vi "Test_Move_Relative.vi"() -> ()   [LabVIEW 2019]
panel:
  in  "Speed input":i16
  in  "Acceleration input":u16
  in  "Relative move distance":i32
  in  "Address":u8
  out "New target":i32
  out "Current position":i32
  in  "COM Port for serial\nconnection. Check device\nmanager.":string
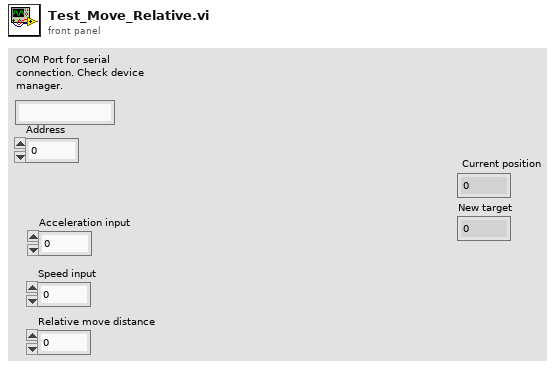
[diagram p1: front panel]
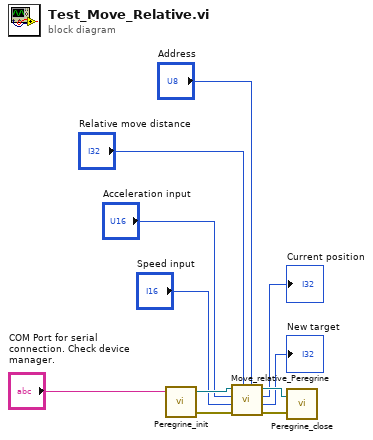
[diagram p0: block diagram]
diagram:
  n1 = call "Peregrine_init.vi"("COM Port for serial\nconnection. Check device\nmanager."="COM Port for serial\nconnection. Check device\nmanager.") -> ("error out"=w10:errorcluster, "Handle out"=w11:refnum<visa-resource-name>)  [unwired: 3 in]
  n2 = call "Move_relative_Peregrine.vi"("Address"="Address", "Relative move distance"="Relative move distance", "error"=w10, "Speed input"="Speed input", "Acceleration input"="Acceleration input", "Handle in"=w11) -> ("error out"=w7:errorcluster, "New target"=→"New target":i32, "Current position"=→"Current position":i32, "Handle out"=w8:refnum<visa-resource-name>)  [unwired: 2 in]
  n3 = call "Peregrine_close.vi"("error in (no error)"=w7, "Handle in"=w8) -> ()  [unwired: 1 in, 1 out]
